vi "generateSystemMessageOutput.vi"(2 "New Message":string, 3 "Old Message":string) -> (1 "System Message Output":string)   [LabVIEW 2013]
doc: "Basic Formatting for System Message Box"
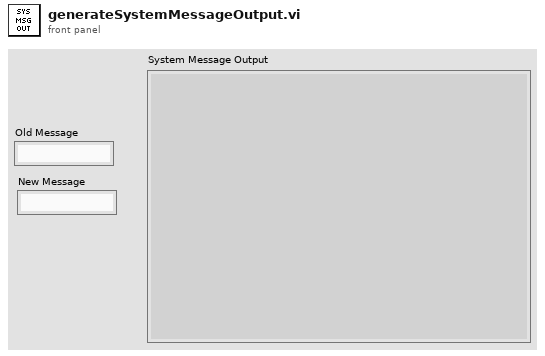
[diagram p1: front panel]
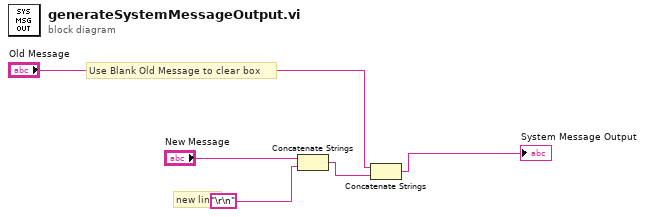
[diagram p0: block diagram]
diagram:
  # "Use Blank Old Message to clear box"
  # "new line"
  n1 = Concatenate Strings("New Message", "\r\n") -> (w4:string)
  n2 = Concatenate Strings("Old Message", w4) -> (→"System Message Output":string)
